vi "Conf Voltage.vi"(0 "VISA Resource Name":refnum<visa-resource-name>, 1 "Set/Check (F:Set)":bool, 2 "Check Parameter (1:Ap Min)":T3(ring)=enum."Aperture Min", 5 "AC/DC (F:DC)":bool, 7 "Autorange? (F:Off)":bool, 9 "Range (6:Max)":T2(ring)=enum."Maximum", 11 "error in (no error)":errorcluster, 12 "Channel List (empty)":string, 13 "Advanced Config":T1={"Aperture Value (.4)"=0.4, "Aperture (1:Minimum)"=1, "NPLC (1)"=2, "Bandwidth (3 Hz)"=0, "Input Impedance (F:Fixed)"=FALSE, "Integration Time (F:Aperture)"=FALSE} {"Bandwidth (3 Hz)" items=["3 Hz", "20 Hz", "200 Hz", "Minimum", "Maximum"]; "NPLC (1)" items=[".02", ".2", "1", "2", "10", "20", "100", "200", "Minimum", "Maximum"]; "Aperture (1:Minimum)" items=["Manual", "Minimum", "Maximum"]; "Aperture Value (.4)" min=0.4 max=4.0 format="%.2f"}) -> (4 "VISA Resource Name Out":refnum<visa-resource-name>, 8 "Configuration?":string, 15 "error out":errorcluster)   [LabVIEW 2012, in "Agilent 34970.lvlib"]
doc: "This VI configures the instrument for advanced voltage measurements.\n\nThis is an advanced measurment configuration VI. For more information on the different ways to take and configure a measurment, refer to the context help and block diagram of \"HP34970A Advanced Scan Example.vi\"."
uses:
  <instrlib>/Agilent 34970/Agilent 34970.lvlib
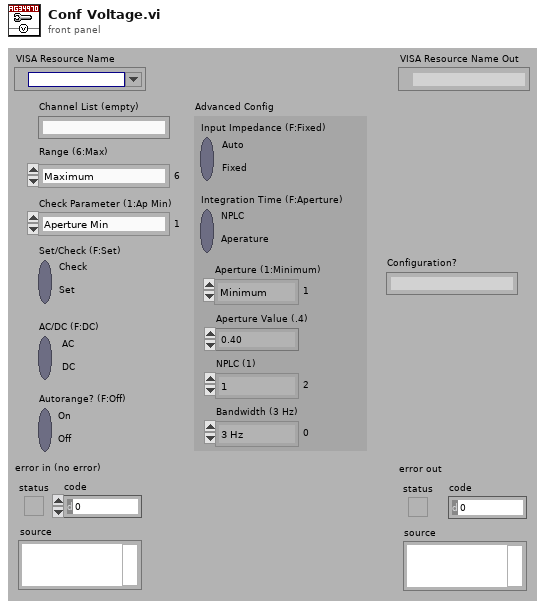
[diagram p1: front panel]
types:
  T1 = cluster{"Aperture Value (.4)":dbl, "Aperture (1:Minimum)":u16, "NPLC (1)":u16, "Bandwidth (3 Hz)":u16, "Input Impedance (F:Fixed)":bool, "Integration Time (F:Aperture)":bool}
  T2 = enum16{"100 mV", "1 V", "10 V", "100 V", "300 V", "Minimum", "Maximum"}
  T3 = enum16{"Aperture (By Chan)", "Aperture Min", "Aperture Max", "NPLC (By Chan)", "NPLC Min", "NPLC Max", "Bandwidth (By Chan)", "Bandwidth Min", "Bandwidth Max", "Impedance (By Chan)"}
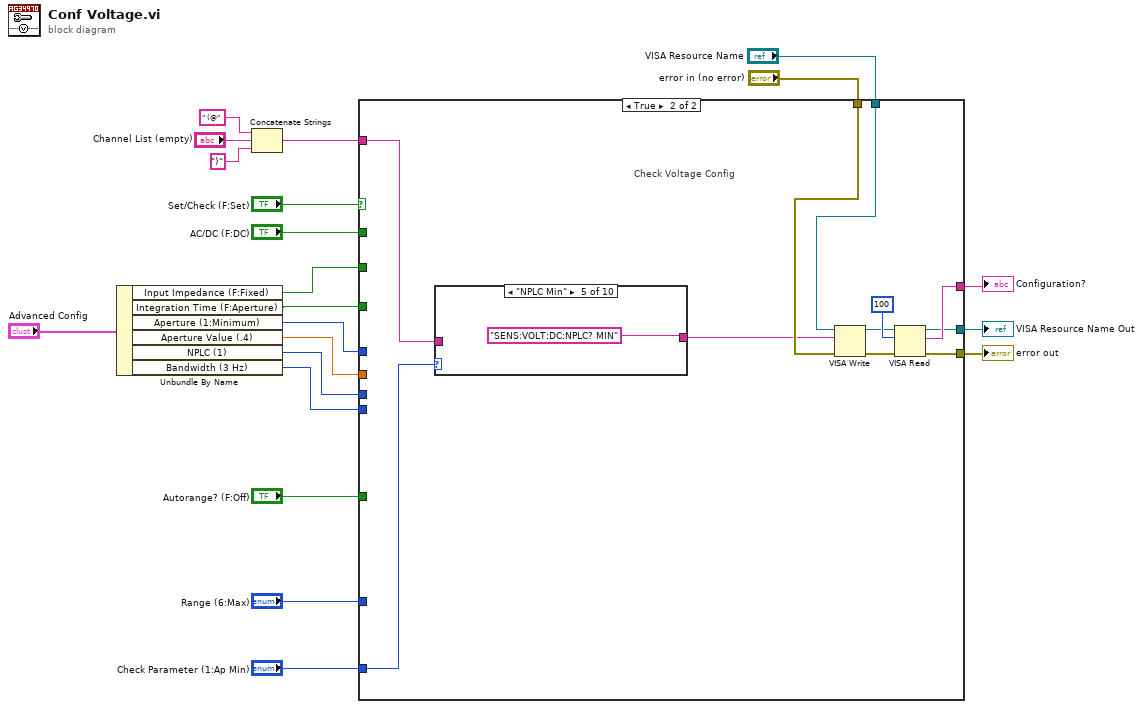
[diagram p0: block diagram]
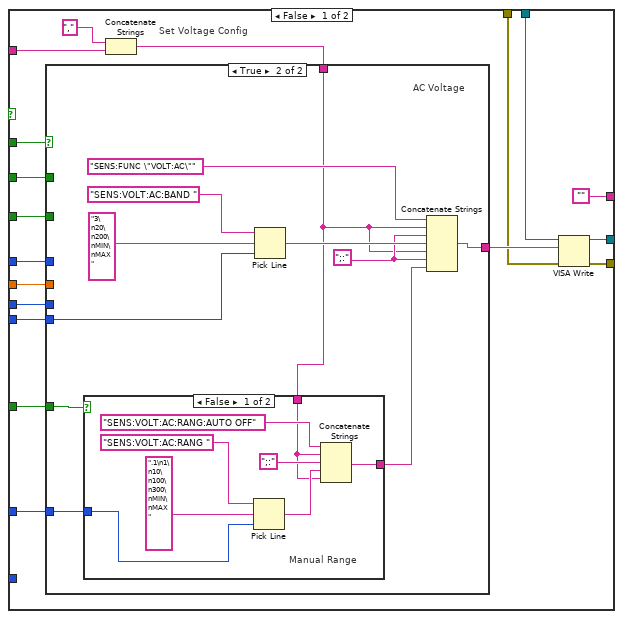
[diagram p2: hidden frame]
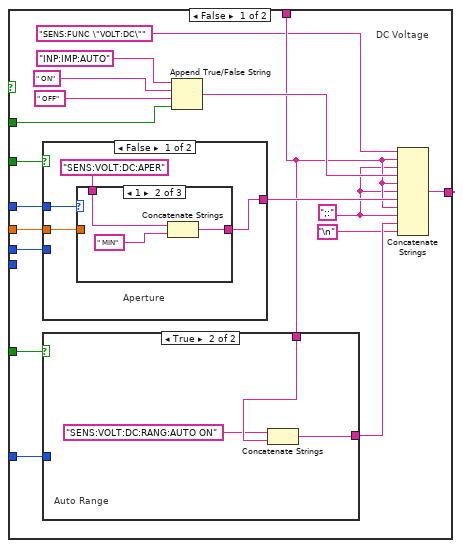
[diagram p3: hidden frame]
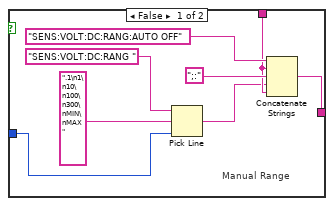
[diagram p4: hidden frame]
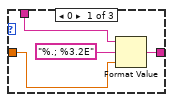
[diagram p5: hidden frame]
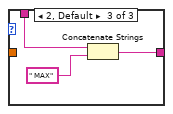
[diagram p6: hidden frame]
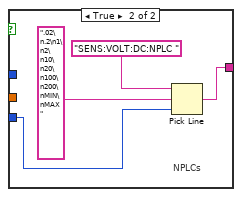
[diagram p7: hidden frame]
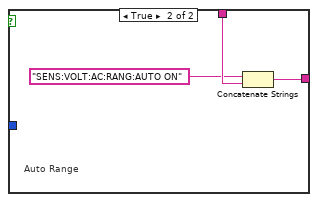
[diagram p8: hidden frame]
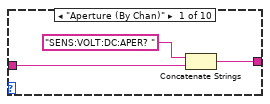
[diagram p9: hidden frame]
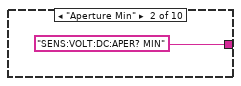
[diagram p10: hidden frame]
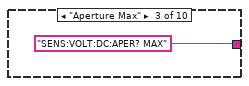
[diagram p11: hidden frame]
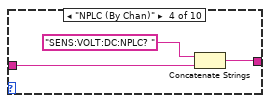
[diagram p12: hidden frame]
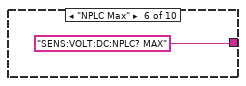
[diagram p13: hidden frame]
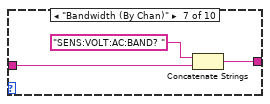
[diagram p14: hidden frame]
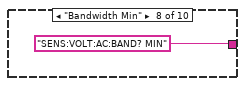
[diagram p15: hidden frame]
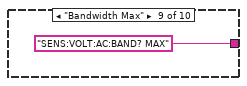
[diagram p16: hidden frame]
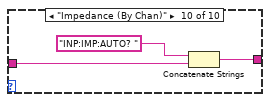
[diagram p17: hidden frame]
diagram:
  n1 = Unbundle By Name("Advanced Config") -> ("Input Impedance (F:Fixed)"=w11:bool, "Integration Time (F:Aperture)"=w10:bool, "Aperture (1:Minimum)"=w9:u16, "Aperture Value (.4)"=w8:dbl, "NPLC (1)"=w7:u16, "Bandwidth (3 Hz)"=w6:u16)
  n2 = Concatenate Strings(" (@", "Channel List (empty)", ")") -> (w16:string)
  n3 = case shown="True" "Set/Check (F:Set)" {
    tunnel: [w28 w119] -> w2
    tunnel: [w29 w116] -> w3
    tunnel: "AC/DC (F:DC)" -> [w39 _]
    tunnel: w11 -> [w38 _]
    tunnel: w9 -> [w37 _]
    tunnel: w8 -> [w36 _]
    tunnel: w7 -> [w35 _]
    tunnel: w16 -> [w34 w112]
    tunnel: w6 -> [w31 _]
    tunnel: ["" w117] -> w15
    tunnel: "Check Parameter (1:Ap Min)" -> [_ w113]
    tunnel: w10 -> [w27 _]
    tunnel: "Autorange? (F:Off)" -> [w26 _]
    tunnel: "Range (6:Max)" -> [w25 _]
    tunnel: "VISA Resource Name" -> [w23 w111]
    tunnel: "error in (no error)" -> [w22 w110]
    frame False {
      # "Set Voltage Config"
      n4 = Concatenate Strings(",", w34) -> (w32:string)
      n5 = case shown="True" w39 {
        tunnel: w38 -> [w56 _]
        tunnel: w37 -> [w49 _]
        tunnel: w36 -> [w50 _]
        tunnel: w35 -> [w48 _]
        tunnel: w32 -> [w44 w87]
        tunnel: w31 -> [_ w89]
        tunnel: [w54 w94] -> w24
        tunnel: w27 -> [w51 _]
        tunnel: w26 -> [w46 w92]
        tunnel: w25 -> [w45 w91]
        frame False {
          w43 = ";:"
          # "DC Voltage"
          n6 = case shown="False" w51 {
            tunnel: w50 -> [w71 _]
            tunnel: w49 -> [w70 _]
            tunnel: w48 -> [_ w84]
            tunnel: [w69 w83] -> w47
            frame False {
              # "Aperture"
              n7 = case shown="1" w70 {
                tunnel: "SENS:VOLT:DC:APER" -> [w76 w79 w81]
                tunnel: [w74 w77 w80] -> w69
                tunnel: w71 -> [w73 _ _]
                frame 0 {
                  n8 = Format Value(string ("")=w76, format string="%.; %3.2E", value (0)=w73) -> (output string=w74:string)
                }
                frame 1 {
                  n9 = Concatenate Strings(w79, " MIN") -> (w77:string)
                }
                frame 2, Default {
                  n10 = Concatenate Strings(w81, " MAX") -> (w80:string)
                }
              }
            }
            frame True {
              # "NPLCs"
              n11 = Pick Line(string ("")="SENS:VOLT:DC:NPLC ", multi-line string=".02\n.2\n1\n2\n10\n20\n100\n200\nMIN\nMAX", line index=w84) -> (output string=w83:string)
            }
          }
          n12 = case shown="True" w46 {
            tunnel: w45 -> [w63 _]
            tunnel: w44 -> [w60 w68]
            tunnel: [w59 w66] -> w42
            frame False {
              # "Manual Range"
              n13 = Pick Line(string ("")="SENS:VOLT:DC:RANG ", multi-line string=".1\n1\n10\n100\n300\nMIN\nMAX", line index=w63) -> (output string=w58:string)
              n14 = Concatenate Strings("SENS:VOLT:DC:RANG:AUTO OFF", w60, ";:", w58, w60) -> (w59:string)
            }
            frame True {
              # "Auto Range"
              n15 = Concatenate Strings("SENS:VOLT:DC:RANG:AUTO ON", w68) -> (w66:string)
            }
          }
          n16 = Append True/False String(1:w56, 2:" OFF", 3:" ON", 4:"INP:IMP:AUTO") -> (0:w55:string)
          n17 = Concatenate Strings("SENS:FUNC \"VOLT:DC\"", w44, w43, w55, w44, w43, w47, w44, w43, w42, "\n") -> (w54:string)
        }
        frame True {
          w88 = ";:"
          # "AC Voltage"
          n18 = case shown="False" w92 {
            tunnel: w91 -> [w103 _]
            tunnel: w87 -> [w99 w108]
            tunnel: [w98 w106] -> w90
            frame False {
              # "Manual Range"
              n19 = Pick Line(string ("")="SENS:VOLT:AC:RANG ", multi-line string=".1\n1\n10\n100\n300\nMIN\nMAX", line index=w103) -> (output string=w100:string)
              n20 = Concatenate Strings("SENS:VOLT:AC:RANG:AUTO OFF", w99, ";:", w100, w99) -> (w98:string)
            }
            frame True {
              # "Auto Range"
              n21 = Concatenate Strings("SENS:VOLT:AC:RANG:AUTO ON", w108) -> (w106:string)
            }
          }
          n22 = Pick Line(string ("")="SENS:VOLT:AC:BAND ", multi-line string="3\n20\n200\nMIN\nMAX", line index=w89) -> (output string=w95:string)
          n23 = Concatenate Strings("SENS:FUNC \"VOLT:AC\"", w87, w88, w95, w87, w88, w90) -> (w94:string)
        }
      }
      n24 = VISA Write(VISA resource name=w23, write buffer=w24, error in (no error)=w22) -> (VISA resource name out=w29:refnum<visa-resource-name>, error out=w28:errorcluster)  [unwired: 1 out]
    }
    frame True {
      # "Check Voltage Config"
      n25 = case shown="\"NPLC Min\"" w113 {
        tunnel: w112 -> [w122 _ _ w126 _ _ w131 _ _ w136]
        tunnel: [w120 "SENS:VOLT:DC:APER? MIN" "SENS:VOLT:DC:APER? MAX" w125 "SENS:VOLT:DC:NPLC? MIN" "SENS:VOLT:DC:NPLC? MAX" w130 "SENS:VOLT:AC:BAND? MIN" "SENS:VOLT:AC:BAND? MAX" w135] -> w109
        frame "Aperture (By Chan)" {
          n26 = Concatenate Strings("SENS:VOLT:DC:APER? ", w122) -> (w120:string)
        }
        frame "Aperture Min" {
        }
        frame "Aperture Max" {
        }
        frame "NPLC (By Chan)" {
          n27 = Concatenate Strings("SENS:VOLT:DC:NPLC? ", w126) -> (w125:string)
        }
        frame "NPLC Min" {
        }
        frame "NPLC Max" {
        }
        frame "Bandwidth (By Chan)" {
          n28 = Concatenate Strings("SENS:VOLT:AC:BAND? ", w131) -> (w130:string)
        }
        frame "Bandwidth Min" {
        }
        frame "Bandwidth Max" {
        }
        frame "Impedance (By Chan)" {
          n29 = Concatenate Strings("INP:IMP:AUTO? ", w136) -> (w135:string)
        }
      }
      n30 = VISA Write(VISA resource name=w111, write buffer=w109, error in (no error)=w110) -> (VISA resource name out=w115:refnum<visa-resource-name>, error out=w114:errorcluster)  [unwired: 1 out]
      n31 = VISA Read(VISA resource name=w115, byte count=u32 100 ("byte count (0)"), error in (no error)=w114) -> (VISA resource name out=w116:refnum<visa-resource-name>, read buffer=w117:string, error out=w119:errorcluster)  [unwired: 1 out]
    }
  }
  "Configuration?" <- w15
  "error out" <- w2
  "VISA Resource Name Out" <- w3
